vi "Get Constants.vi"() -> (4 "constants":T1)   [LabVIEW 2019]
uses:
  TypeDefs/Constants.ctl
  Global Constants.vi
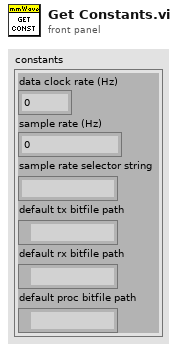
[diagram p1: front panel]
types:
  T1 = typedef "Constants.ctl" = cluster{"data clock rate (Hz)":dbl, "sample rate (Hz)":dbl, "sample rate selector string":string, "default tx bitfile path":path, "default rx bitfile path":path, "default proc bitfile path":path}
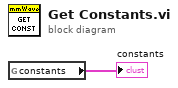
[diagram p0: block diagram]
diagram:
  n1 = global read "Global Constants.vi" "constants"() -> (→"constants":T1)
